vi "Configure Measurement.vi"(6 "Manual Range (1)":dbl=1.0, 7 "Absolute Resolution (1E-6)":dbl=1e-06, 8 "error in (no error)":errorcluster, 9 "Auto Range (T: Enable)":bool=TRUE, 10 "Measurement Function (10: Voltage DC)":i32(ring)=10 items=["Continuity", "Current AC", "Current DC", "Diode", "Frequency", "Resistance 4-wire", "Period", "Resistance 2-wire", "Temperature", "Voltage AC", "Voltage DC", "Voltage DC Ratio", "Capacitance"], 11 "VISA resource name":refnum<visa-resource-name>) -> (0 "error out":errorcluster, 3 "VISA resource name out":refnum<visa-resource-name>)   [LabVIEW 2023, in "Agilent 3446X Series.lvlib"]
doc: "Configures the measurement type, resolution, and range on the instrument."
uses:
  Agilent 3446X Series.lvlib
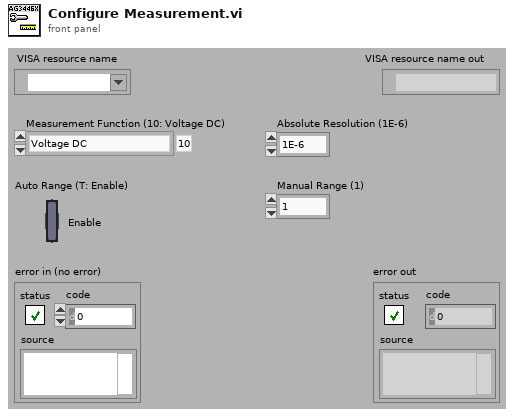
[diagram p1: front panel]
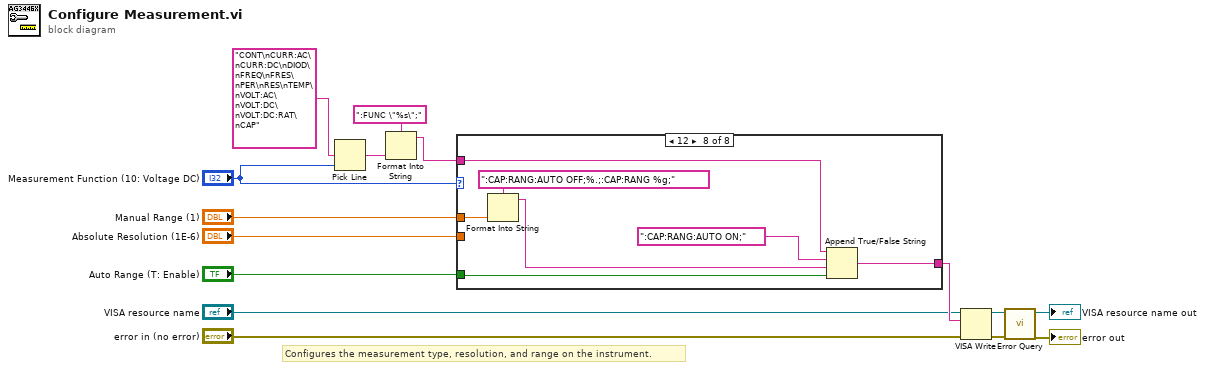
[diagram p0: block diagram]
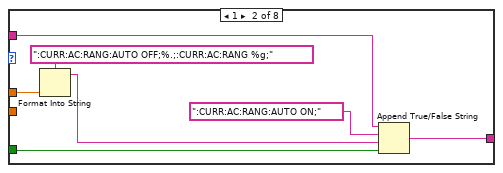
[diagram p3: hidden frame]
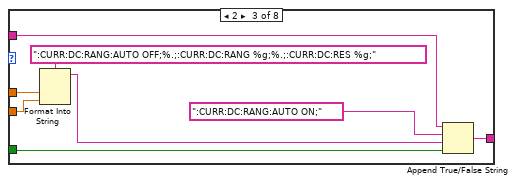
[diagram p4: hidden frame]
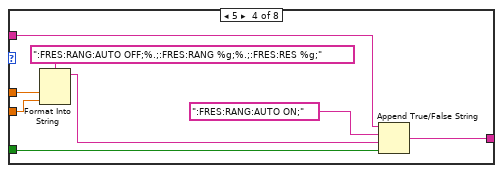
[diagram p5: hidden frame]
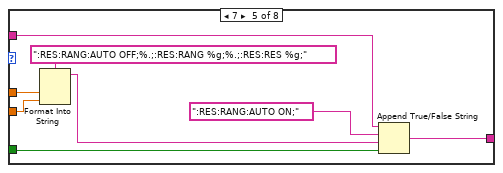
[diagram p6: hidden frame]
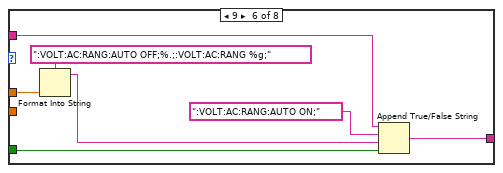
[diagram p7: hidden frame]
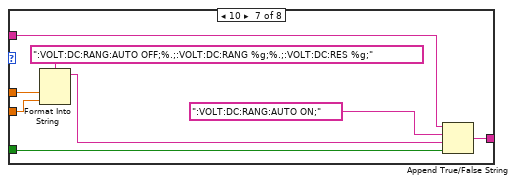
[diagram p8: hidden frame]
diagram:
  # "Configures the measurement type, resolution, and range on the instrument."
  n1 = Pick Line(multi-line string="CONT\nCURR:AC\nCURR:DC\nDIOD\nFREQ\nFRES\nPER\nRES\nTEMP\nVOLT:AC\nVOLT:DC\nVOLT:DC:RAT\nCAP", line index="Measurement Function (10: Voltage DC)") -> (output string=w4:string)  [unwired: 1 out]
  n2 = Format Into String(format string=":FUNC \"%s\";", w4) -> (resulting string=w5:string)  [unwired: 2 in, 1 out]
  n3 = case shown="12" "Measurement Function (10: Voltage DC)" {
    tunnel: "Auto Range (T: Enable)" -> [_ w20 w28 w36 w44 w51 w58 w66]
    tunnel: w5 -> [w16 w19 w27 w35 w43 w50 w59 w65]
    tunnel: [w16 w18 w25 w33 w42 w49 w56 w64] -> w3
    tunnel: "Absolute Resolution (1E-6)" -> [_ _ w26 w34 w41 _ w57 _]
    tunnel: "Manual Range (1)" -> [_ w17 w24 w32 w40 w48 w55 w63]
    frame 0, 3, 4, 6, 8, 11, Default {
    }
    frame 1 {
      n4 = Format Into String(format string=":CURR:AC:RANG:AUTO OFF;%.;:CURR:AC:RANG %g;", w17) -> (resulting string=w21:string)  [unwired: 2 in, 1 out]
      n5 = Append True/False String(1:w20, 2:w21, 3:":CURR:AC:RANG:AUTO ON;", 4:w19) -> (0:w18:string)
    }
    frame 2 {
      n6 = Format Into String(format string=":CURR:DC:RANG:AUTO OFF;%.;:CURR:DC:RANG %g;%.;:CURR:DC:RES %g;", w24, w26) -> (resulting string=w29:string)  [unwired: 2 in, 1 out]
      n7 = Append True/False String(1:w28, 2:w29, 3:":CURR:DC:RANG:AUTO ON;", 4:w27) -> (0:w25:string)
    }
    frame 5 {
      n8 = Format Into String(format string=":FRES:RANG:AUTO OFF;%.;:FRES:RANG %g;%.;:FRES:RES %g;", w32, w34) -> (resulting string=w37:string)  [unwired: 2 in, 1 out]
      n9 = Append True/False String(1:w36, 2:w37, 3:":FRES:RANG:AUTO ON;", 4:w35) -> (0:w33:string)
    }
    frame 7 {
      n10 = Format Into String(format string=":RES:RANG:AUTO OFF;%.;:RES:RANG %g;%.;:RES:RES %g;", w40, w41) -> (resulting string=w45:string)  [unwired: 2 in, 1 out]
      n11 = Append True/False String(1:w44, 2:w45, 3:":RES:RANG:AUTO ON;", 4:w43) -> (0:w42:string)
    }
    frame 9 {
      n12 = Format Into String(format string=":VOLT:AC:RANG:AUTO OFF;%.;:VOLT:AC:RANG %g;", w48) -> (resulting string=w52:string)  [unwired: 2 in, 1 out]
      n13 = Append True/False String(1:w51, 2:w52, 3:":VOLT:AC:RANG:AUTO ON;", 4:w50) -> (0:w49:string)
    }
    frame 10 {
      n14 = Format Into String(format string=":VOLT:DC:RANG:AUTO OFF;%.;:VOLT:DC:RANG %g;%.;:VOLT:DC:RES %g;", w55, w57) -> (resulting string=w60:string)  [unwired: 2 in, 1 out]
      n15 = Append True/False String(1:w58, 2:w60, 3:":VOLT:DC:RANG:AUTO ON;", 4:w59) -> (0:w56:string)
    }
    frame 12 {
      n16 = Format Into String(format string=":CAP:RANG:AUTO OFF;%.;:CAP:RANG %g;", w63) -> (resulting string=w67:string)  [unwired: 2 in, 1 out]
      n17 = Append True/False String(1:w66, 2:w67, 3:":CAP:RANG:AUTO ON;", 4:w65) -> (0:w64:string)
    }
  }
  n18 = VISA Write(VISA resource name="VISA resource name", write buffer=w3, error in (no error)="error in (no error)") -> (VISA resource name out=w13:refnum<visa-resource-name>, error out=w12:errorcluster)  [unwired: 1 out]
  n19 = call "Error Query.vi"("error in (no error)"=w12, "VISA resource name"=w13) -> ("error out"=→"error out":errorcluster, "VISA resource name out"=→"VISA resource name out":refnum<visa-resource-name>)  [unwired: 8 out]
